vi "Actor Core.vi"(8 "error in":errorcluster, 11 "MFC Actor.lvlib:MFC.lvclass":refnum<class "Scale.lvclass">) -> (0 "error out":errorcluster, 3 "Actor out":refnum<class "Actor.lvclass">)   [LabVIEW 2013, in "Scale.lvlib" / "Scale.lvclass"]
doc: "This is Actor Core.vi, the main message handling loop for Actors. An actor usually just sits in this loop and processes messages as they arrive. Any error returned by the message Do.vi call will stop the loop, with error code 43 as the canonical signal to stop with no error sent to caller. Descendants may override that in Handle Error.vi."
uses:
  Scale.lvclass
  PluginInterface/Actor Framework.lvlibp/Actor/Actor.lvclass
  Scale.lvclass/Scale.ctl
  PluginInterface/PluginInterface.lvlibp/PluginInterfaceClass/PluginInterface.lvclass
  Write Graph.vi
  Write Value.vi
  Write Graph History.vi
  PluginInterface/PluginInterface.lvlibp/PluginInterfaceClass/Write VI Refnum.vi
  PluginInterface/Actor Framework.lvlibp/Message Enqueuer/Enqueue.vi
  Scale Messages/Initialize Msg/Initialize Msg.lvclass
  Scale Messages/Update Graphs Msg/Update Graphs Msg.lvclass
  Scale Messages/Read Scale Msg/Read Scale Msg.lvclass
  Scale Messages/Log Data Msg/Log Data Msg.lvclass
  PluginInterface/Actor Framework.lvlibp/Stop Msg/Stop Msg.lvclass
panel:
  in  "stop signal":bool
  in  "Round Color Box 3":u32(colorbox)=483491
  out "Value 1":dbl=36.53012927910604
  in  "Graph History":dbl=300.0
  out "Graph 2":T1(graph) caption="Pump A"
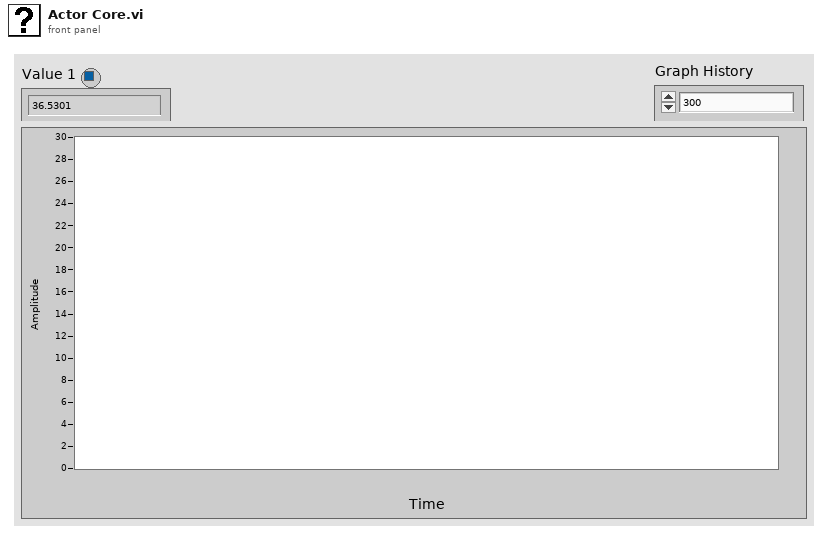
[diagram p1: front panel]
types:
  T1 = cluster{"output array":dbl[], "output array":dbl[]}
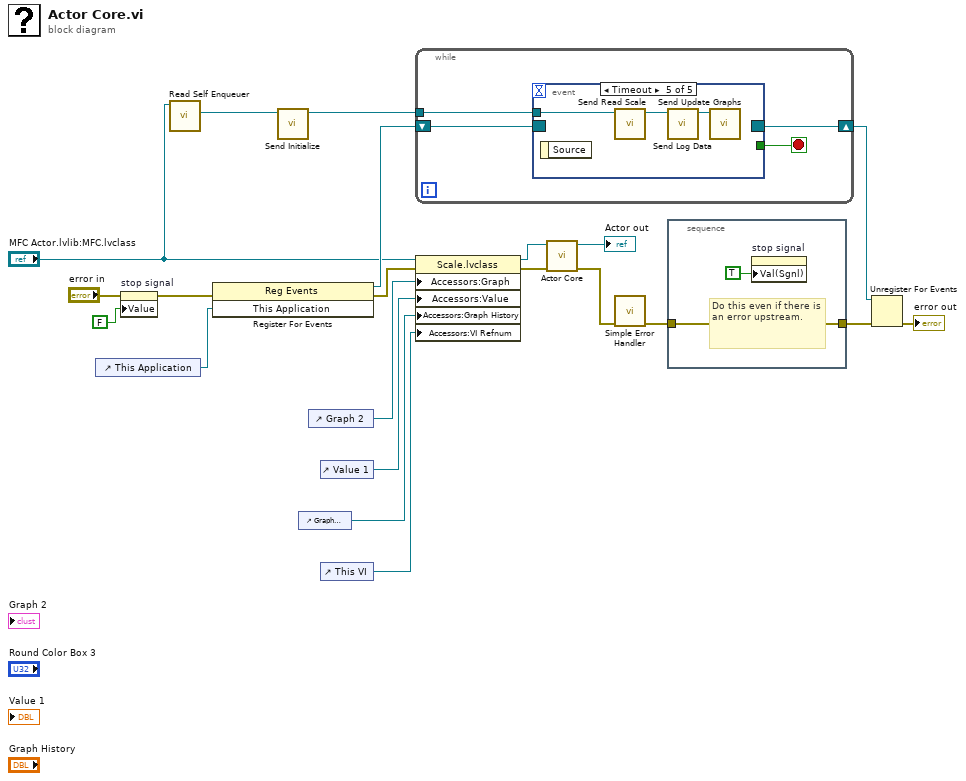
[diagram p0: block diagram]
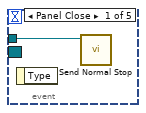
[diagram p2: hidden frame]
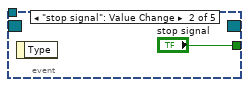
[diagram p3: hidden frame]
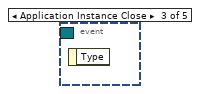
[diagram p4: hidden frame]
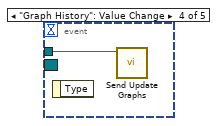
[diagram p5: hidden frame]
diagram:
  n1 = control-ref of="This Application"() -> (w14:refnum<vi>)
  n2 = property on="stop signal" class="Bool (strict)"(error in="error in", "Value"=FALSE ("stop")) -> (error out=w15:errorcluster)  [unwired: 1 in, 1 out]
  n3 = call "Read Self Enqueuer.vi"("Actor"="MFC Actor.lvlib:MFC.lvclass") -> ("Self Enqueuer"=w8:refnum<class "Message Enqueuer.lvclass">)  [unwired: 10 in]
  n4 = register-events(error in=w15, w14) -> (reference out=w18:refnum<event-registration>, error out=w2:errorcluster)  [unwired: 1 in]
  n5 = call "Send Initialize.vi"("Message Enqueuer"=w8) -> ("Message Enqueuer out"=w3:refnum<class "Message Enqueuer.lvclass">)  [unwired: 9 in, 1 out]
  n6 = control-ref of="Graph History"() -> (w5:refnum<vi>)
  n7 = control-ref of="Graph 2"() -> (w4:refnum<vi>)
  n8 = control-ref of="Value 1"() -> (w7:refnum<vi>)
  n9 = control-ref of="This VI"() -> (w1:refnum<vi>)
  n10 = while {
    tunnel: w3 -> [w25]
    shift-right: [w22] -> w17
    shift-left: w18 -> [w23]
    stop <- w24 stop-if-true
    n11 = event shown="[4] Timeout" {
      selector: w23 -> [_ _ _ _ _]
      dyn-events: [_ _ _ _ _] -> w22
      timeout: _ -> [_ _ _ _ _]
      tunnel: w25 -> [w26 _ _ w28 w31]
      tunnel: [_ "stop signal" _ _ _] -> w24
      event Panel Close {
        n12 = event-data() -> ()  [unwired: 1 in, 1 out]
        n13 = call "Send Normal Stop.vi"("Message Enqueuer"=w26) -> ()  [unwired: 10 in, 1 out]
      }
      event "stop signal": Value Change {
        n14 = event-data() -> ()  [unwired: 1 in, 1 out]
      }
      event Application Instance Close {
        n15 = event-data() -> ()  [unwired: 1 in, 1 out]
      }
      event "Graph History": Value Change {
        n16 = event-data() -> ()  [unwired: 1 in, 1 out]
        n17 = call "Send Update Graphs.vi"("Message Enqueuer"=w28) -> ()  [unwired: 9 in, 2 out]
      }
      event Timeout {
        n18 = event-data() -> ()  [unwired: 1 in, 1 out]
        n19 = call "Send Read Scale.vi"("Message Enqueuer"=w31) -> ("Message Enqueuer out"=w29:refnum<class "Message Enqueuer.lvclass">)  [unwired: 9 in, 1 out]
        n20 = call "Send Log Data.vi"("Message Enqueuer"=w29) -> ("Message Enqueuer out"=w30:refnum<class "Message Enqueuer.lvclass">)  [unwired: 9 in, 1 out]
        n21 = call "Send Update Graphs.vi"("Message Enqueuer"=w30) -> ()  [unwired: 9 in, 2 out]
      }
    }
  }
  n22 = property class="Scale.lvclass"(reference="MFC Actor.lvlib:MFC.lvclass", error in=w2, "Accessors:Graph"=w4, "Accessors:Value"=w7, "Accessors:Graph History"=w5, "Accessors:VI Refnum"=w1) -> (reference out=w13:refnum<class "Scale.lvclass">, error out=w9:errorcluster)
  n23 = call-parent "Actor Core.vi"("error in"=w9, "Actor in"=w13) -> ("error out"=w20:errorcluster, "Actor out"=→"Actor out":refnum<class "Actor.lvclass">)  [unwired: 8 in]
  n24 = call <vilib>:"Simple Error Handler.vi"("error in (no error)"=w20) -> ("error out"=w19:errorcluster)  [unwired: 4 in, 4 out]
  n25 = stacked-sequence {
    tunnel: [w32] -> w16
    tunnel: w19 -> [w32]
    frame #0 {
      # "Do this even if there is an error upstream."
      n26 = property on="stop signal" class="Bool (strict)"("Val(Sgnl)"=TRUE ("stop")) -> ()  [unwired: 2 in, 2 out]
    }
  }
  n27 = Unregister For Events(event registration refnum=w17, error in=w16) -> (error out=→"error out":errorcluster)
